vi "CMD_Reset.vi"(1 "Line":string) -> (0 "Done":bool)   [LabVIEW 2014]
uses:
  Robot Global Data.vi
  navX-MXP Library/navX-MXP IMU.lvlib
panel:
  in  "Parameters":i32[](array[numeric])=[0, 1, 0]
  in  "Subcommands":string[](array[string])=["gyro", "gyro", "encoders"]
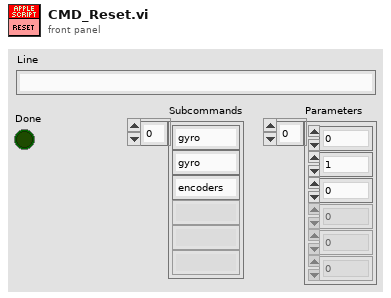
[diagram p1: front panel]
types:
  T1 = typedef "navX-MXP IMU.lvlib/navX SPI DevRef.ctl" = cluster{"SPIDevRef":T2, "Board Information":T5, "Status":T6, "Offsets":cluster{"Yaw":dbl, "Quat W":dbl, "Quat X":dbl, "Quat Y":dbl, "Quat Z":dbl}, "Update Rate (4Hz-60Hz)":u8, "refnum name":string, "error":errorcluster}
  T2 = typedef "WPI_SPIDevRef.ctl" = cluster{"DevStatus":errorcluster, "Handle":i32, "Controller":T3, "SPI Bus":T4}
  T3 = typedef "FPGA_TypedefDigitalModule.ctl" = enum16{"Controller 1"}
  T4 = typedef "spi_bus.ctl" = enum16{"SPI On-Board, CS0", "SPI On-Board, CS1", "SPI On-Board, CS2", "SPI On-Board, CS3", "SPI MXP", "Invalid"}
  T5 = typedef "navX-MXP IMU.lvlib/navX Board Information.ctl" = cluster{"WhoAmI (50 | 0x32)":u8, "Board Revision":u8, "Firmware Major Version":u8, "Firmware Minor Version":u8}
  T6 = typedef "navX-MXP IMU.lvlib/navX Status Data.ctl" = cluster{"Update Rate Hz":u8, "Accelerometer Full-Scale Range":u8, "Gyro Full-Scale Range":u16, "NAVX_OP_STATUS":T7, "NAVX_CAL_STATUS":T8, "NAVX_SELFTEST_STATUS":u8, "NAVX_SENSOR_STATUS":T9}
  T7 = typedef "navX-MXP IMU.lvlib/navX NAVX_OP_STATUS.ctl" = u8
  T8 = typedef "navX-MXP IMU.lvlib/navX NAVX_CAL_STATUS.ctl" = u8
  T9 = typedef "navX-MXP IMU.lvlib/navX NAVX_SENSOR_STATUS.ctl" = cluster{"MOVING":bool, "YAW_STABLE":bool, "MAG_DISTURBANCE":bool, "ALTITUDE_VALID":bool, "SEALEVEL_PRESS_SET":bool, "FUSED_HEADING_VALID":bool}
  T10 = typedef "navX-MXP IMU.lvlib/navX YPRH Data.ctl" = cluster{"Yaw":dbl, "Pitch":dbl, "Roll":dbl, "Heading":dbl}
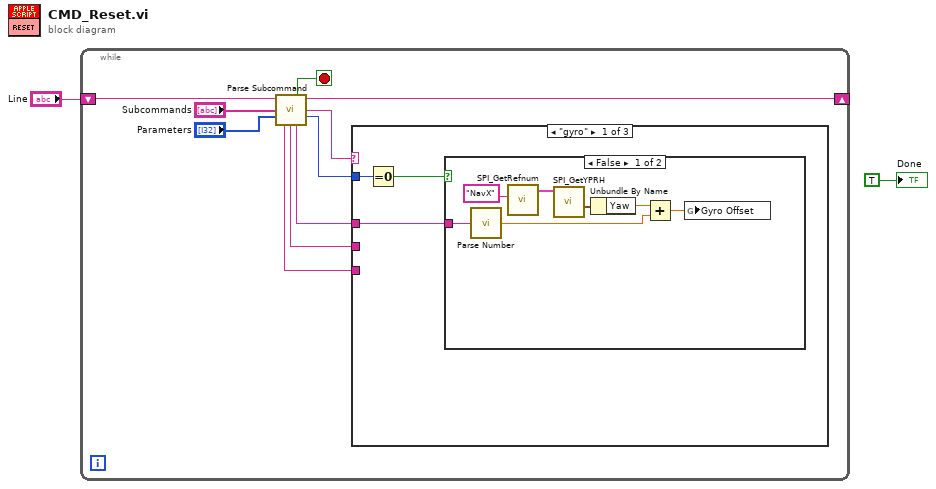
[diagram p0: block diagram]
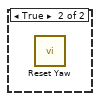
[diagram p2: hidden frame]
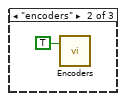
[diagram p3: hidden frame]
diagram:
  n1 = while {
    shift-right: [w9] -> _
    shift-left: "Line" -> [w12]
    stop <- w8 stop-if-true
    n2 = call "Parse Subcommand.vi"("Text In"=w12, "Subcommands"="Subcommands", "Parameters"="Parameters") -> ("Done"=w8:bool, "Text Out"=w9:string, "Subcommand"=w7:string, "# of Parameters"=w6:i32, "Parameter 3"=w3:string, "Parameter 2"=w4:string, "Parameter 1"=w5:string)  [unwired: 6 in]
    n3 = case shown="\"gyro\"" w7 {
      tunnel: w6 -> [w15 _ _]
      tunnel: w5 -> [w13 _ _]
      tunnel: w4 -> [_ _ _]
      tunnel: w3 -> [_ _ _]
      frame "gyro" {
        n4 = Equal To 0?(x=w15) -> (x = 0?=w14:bool)
        n5 = case shown="False" w14 {
          tunnel: w13 -> [w22 _]
          frame False {
            n6 = call "Parse Number.vi"("String"=w22) -> ("Number"=w17:dbl)
            n7 = call "SPI_GetRefnum.vi"("refnum name"="NavX") -> ("navX DevRef"=w19:T1)  [unwired: 9 in, 1 out]
            n8 = call "SPI_GetYPRH.vi"("navX DevRef"=w19) -> ("YPRH"=w20:T10)  [unwired: 8 in, 2 out]
            n9 = Unbundle By Name(w20) -> ("Yaw"=w18:dbl)
            n10 = Add(x=w18, y=w17) -> (x+y=w16:dbl)
            n11 = global write "Robot Global Data.vi" "Gyro Offset"(w16) -> ()
          }
          frame True {
            n12 = call "Reset Yaw.vi"() -> ()  [unwired: 12 in]
          }
        }
      }
      frame "encoders" {
        n13 = call "Encoders.vi"("Reset All"=TRUE) -> ()  [unwired: 1 in, 2 out]
      }
      frame Default {
        # "If subcommand not recognized"
      }
    }
  }
  "Done" <- TRUE
